vi "Check XML File against XSD Schema.vi"(8 "error in (no error)":errorcluster, 10 "XML Configuration File Path":path=path "E:/Ballard - Arinc-429 CD/Example Database/Ballard/XML_000.XML", 11 "XML Schema File Path":path=path "E:/Ballard - Arinc-429 CD/Source/System Explorer/SubVIs/Parse XML Ballard/BTI.XSD") -> (0 "error IO":errorcluster)   [LabVIEW 2020, in "Ballard 1553 System Explorer.lvlib"]
uses:
  Ballard 1553 System Explorer.lvlib
  C:/Users/Administrator/Desktop/GIT/Ballard-MIL-STD-1553-Custom-Device/Source/System Explorer/SubVIs/Parse XML Ballard/1.2/BTIXML_SerDes.dll
  1.2/BTIXML_SerDes.dll
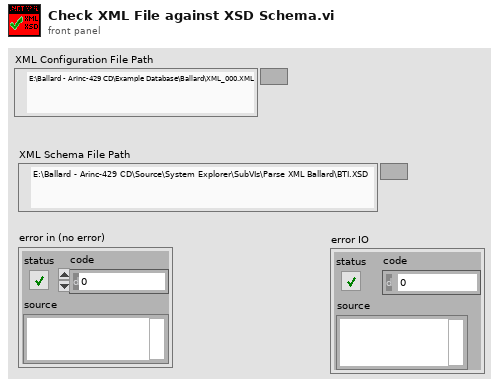
[diagram p1: front panel]
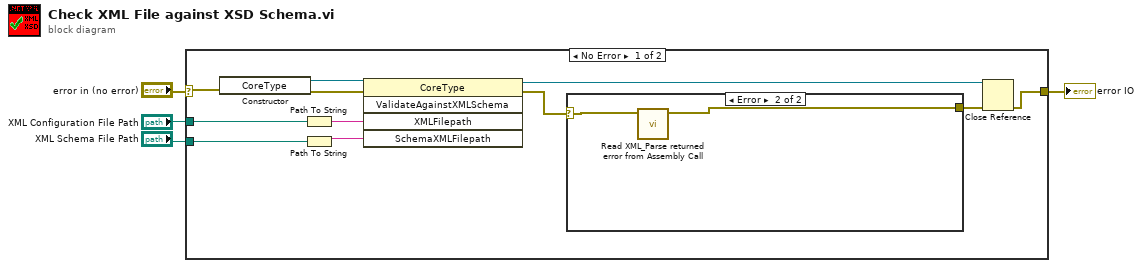
[diagram p0: block diagram]
diagram:
  n1 = case shown="No Error" "error in (no error)" {
    selector: "error in (no error)" -> [w5 w19]
    tunnel: "XML Configuration File Path" -> [w15 _]
    tunnel: "XML Schema File Path" -> [w14 _]
    tunnel: [w12 w19] -> w1
    frame No Error {
      n2 = constructor class="CoreType"(error in=w5) -> (reference out=w7:refnum<k24>, error out=w6:errorcluster)  [unwired: 2 in, 1 out]
      n3 = Path To String(path=w15) -> (string=w8:string)
      n4 = Path To String(path=w14) -> (string=w9:string)
      n5 = invoke class="CoreType" method="ValidateAgainstXMLSchema"(reference=w7, error in=w6, "XMLFilepath"=w8, "SchemaXMLFilepath"=w9) -> (reference out=w11:refnum<k24>, error out=w10:errorcluster)  [unwired: 1 in, 3 out]
      n6 = case shown="Error" w10 {
        selector: w10 -> [w16 w18]
        tunnel: [w16 w17] -> w13
        frame No Error {
        }
        frame Error {
          n7 = call "Read XML_Parse returned error from Assembly Call.vi"("error in (no error)"=w18) -> ("error out"=w17:errorcluster)  [unwired: 10 in]
        }
      }
      n8 = Close Reference(reference=w11, error in (no error)=w13) -> (error out=w12:errorcluster)
    }
    frame Error {
    }
  }
  "error IO" <- w1
